vi "题目4.vi"() -> ()   [LabVIEW 2017]
uses:
  <vilib>/Analysis/2dsp.llb/Real FFT.vi
  <vilib>/Analysis/NI_AALPro.lvlib
  <vilib>/measure/NI_MABase.lvlib
panel:
  in  "sampling info":cluster{"Fs":dbl, "#s":dbl}={"Fs"=1000.0, "#s"=1000.0} caption="采样信息" {"Fs" format="%.2p"}
  in  "幅值3":dbl
  in  "频率3":dbl
  in  "幅值2":dbl
  in  "频率2":dbl
  in  "幅值1":dbl
  in  "频率1":dbl
  out "频域信号":dbl[](graph)
  out "时域信号":dbl[](graph)
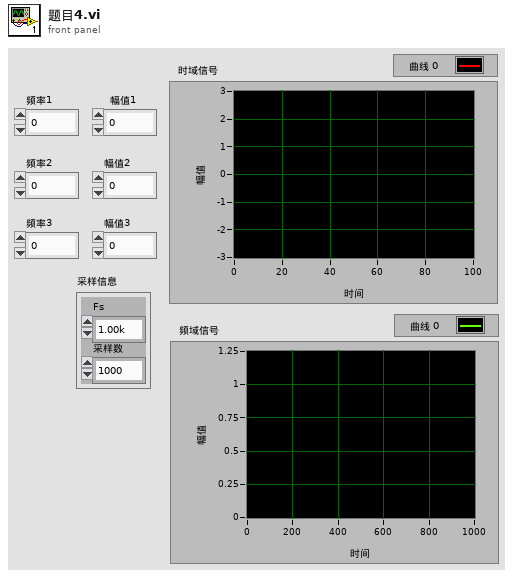
[diagram p1: front panel]
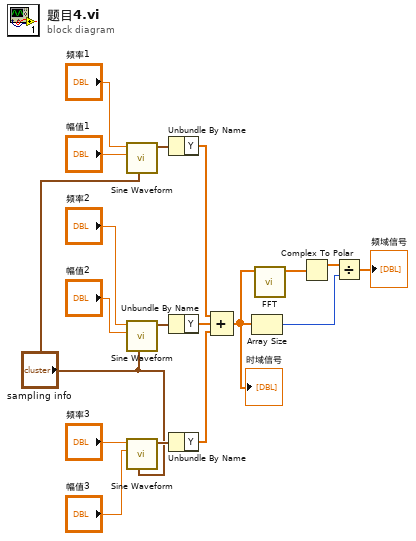
[diagram p0: block diagram]
diagram:
  n1 = call <vilib>:"Sine Waveform.vi"("sampling info"="sampling info", "amplitude"="幅值1", "frequency"="频率1") -> ("signal out"=w16:waveform(dbl))  [unwired: 7 in, 1 out]
  n2 = call <vilib>:"Sine Waveform.vi"("sampling info"="sampling info", "amplitude"="幅值2", "frequency"="频率2") -> ("signal out"=w15:waveform(dbl))  [unwired: 7 in, 1 out]
  n3 = call <vilib>:"Sine Waveform.vi"("sampling info"="sampling info", "amplitude"="幅值3", "frequency"="频率3") -> ("signal out"=w14:waveform(dbl))  [unwired: 7 in, 1 out]
  n4 = Unbundle By Name(w16) -> ("Y"=w13:dbl[])
  n5 = Unbundle By Name(w15) -> ("Y"=w12:dbl[])
  n6 = Unbundle By Name(w14) -> ("Y"=w11:dbl[])
  n7 = Compound Arithmetic op=ADD(w13, w12, w11) -> (w10:dbl[])
  "时域信号" <- w10
  n8 = Array Size(array=w10) -> (size(s)=w17:i32)
  n9 = call-poly <vilib>:"FFT.vi"("X"=w10) -> ("FFT {X}"=w8:cdb[])  [unwired: 9 in, 1 out]
  n10 = Complex To Polar(r * e^(i*theta)=w8) -> (r=w18:dbl[])  [unwired: 1 out]
  n11 = Divide(x=w18, y=w17) -> (x/y=→"频域信号":dbl[])
